vi "Top_Level.vi"() -> ()   [LabVIEW 2013]
uses:
  Classes/OSSP_Problem.lvclass
  Classes/GA.lvclass
  Classes/GA_Class/Controls/Strategy.ctl
  Classes/GA_Class/Controls/Plot Type.ctl
  Classes/GA_Class/Controls/Crossover Type.ctl
  Classes/GA_Class/Controls/Mutation Type.ctl
  Controls/Local Search Type.ctl
  Controls/Problem Instance Type.ctl
  Controls/Scheduler Type.ctl
  Controls/Objective.ctl
  Classes/SA_Class/Controls/Perturbation Method.ctl
  Controls/States.ctl
  Classes/OSSP_Problem.lvclass/OSSP_Problem.ctl
  Classes/GA_Class/Controls/Front Panle Menu.ctl
  Classes/GA.lvclass/GA.ctl
  Controls/SA Solution Selection Method.ctl
  Classes/SA.lvclass/SA.ctl
  Classes/GA_Class/Select Random Solutions.vi
  Classes/GanntChart_Class/Non Delay Scheduler For Tardiness.vi
  Classes/SA_Class/Setters/Write Alpha Value.vi
  Classes/SA_Class/Setters/Write Current Temperature.vi
  Classes/SA_Class/Setters/Write Cooling Strategy.vi
  Classes/SA_Class/Setters/Write Initial Temperature.vi
  Classes/SA_Class/Setters/Write Stop Temperature.vi
  Classes/SA_Class/Setters/Write Cooling Rate.vi
  Classes/SA_Class/Setters/Write Epoch Length.vi
  Classes/SA_Class/Setters/Write Current Solution.vi
  Classes/SA_Class/Setters/Write Best Solution.vi
  Classes/GanntChart_Class/Giffler Thompson Active Schedule Engine.vi
  Classes/GanntChart_Class/Schedule and Create Gannt Chart.vi
  Classes/GanntChart_Class/Calculate Makespan.vi
  Classes/GanntChart_Class/Job Completion Times.vi
  Classes/GanntChart_Class/Reorder Chromosome  After Makespan Calculation.vi
  Classes/SA_Class/Getters/Read Current Solution.vi
  Classes/SA_Class/Setters/Write New Solution.vi
  Classes/SA_Class/Getters/Read New Solution.vi
  Classes/SA_Class/Calculate Acceptance Probability.vi
  Classes/SA_Class/Getters/Read Best Solution.vi
  Classes/SA_Class/Getters/Read Epoch Length.vi
  Classes/SA_Class/Getters/Read Current Temperature.vi
  Classes/SA_Class/Getters/Read Cooling Strategy.vi
  Classes/SA_Class/Getters/Read Cooling Rate.vi
  Classes/SA_Class/Getters/Read Alpha Value.vi
  Classes/SA_Class/Getters/Read Stop Temperature.vi
  Classes/GA_Class/Getters/Read Scheduler.vi
  Classes/GA_Class/Getters/Read Objective .vi
  Classes/GA_Class/Getters/Read Reorder.vi
  Classes/GA_Class/Find Best Solution In Population.vi
  Classes/GanntChart_Class/Operation to Machine Job Tuple.vi
  Classes/GanntChart_Class/Check Other Machines for Schedule Time.vi
  Classes/GanntChart_Class/Schedule Job.vi
  Classes/GanntChart_Class/Find Gaps on Particular Machine.vi
  Classes/GanntChart_Class/Increment Number of Jobs on Machine.vi
  Classes/GanntChart_Class/Find Job On Other Machines.vi
  <vilib>/Analysis/baseanly.llb/Mean (DBL).vi
  Classes/SA_Class/Perturb Current Solution.vi
  Classes/SA.lvclass
  <vilib>/Analysis/NI_AALBase.lvlib
panel:
  out "Makespan":dbl format="%#_13g"
  out "Total Tardiness":i32
  in  "Local Search Per Generation":i32=25
  in  "Perturbation Method":T1
  in  "Local Search":T2
  out "Final Solution":string
  out "Generations":i32(slide) scale=0.0..1001.0
  out "Picture":picture
  in  "Objective":T3=enum."Total Tardiness"
  in  "Reorder":bool=TRUE
  in  "Scheduler":T4=enum."FIFO Scheduler"
  in  "Instance Type":T5=enum."Brucker"
  in  "Mutation Type":T6
  in  "Crossover Type":T7=enum."Linear Order Cx (LOX)"
  in  "Plot Type":T8=enum."Gannt Chart"
  in  "Strategy":T9=enum."Incremental Replacement"
  in  "Number of Generations":i32=1000
  in  "Population Size":u8=30
  in  "Mutation Probability":dbl=0.2
  in  "Crossover Probability":dbl=1.0
  out "Mo4J":u16[][](array[numeric])
  out "JO4M":u16[][](array[numeric])
  out "Due Dates":u16[](array[numeric])
  out "Job Completion Times":u16[](array[numeric])
  out "Job Schedule on Machine":i32[][](array[numeric])
  out "GA.lvclass":refnum<class "GA.lvclass">
  out "OSSP_Problem.lvclass":refnum<class "OSSP_Problem.lvclass">
  out "error out":errorcluster
  in  "error in":errorcluster
  # "Processing tImes =   J1       J2    J3       J4   \n                         M1    X        X      X        X\n                         M2    X        X      X        X\n                         M3    X        X      X        X\n                         M4    X        X      X        X"
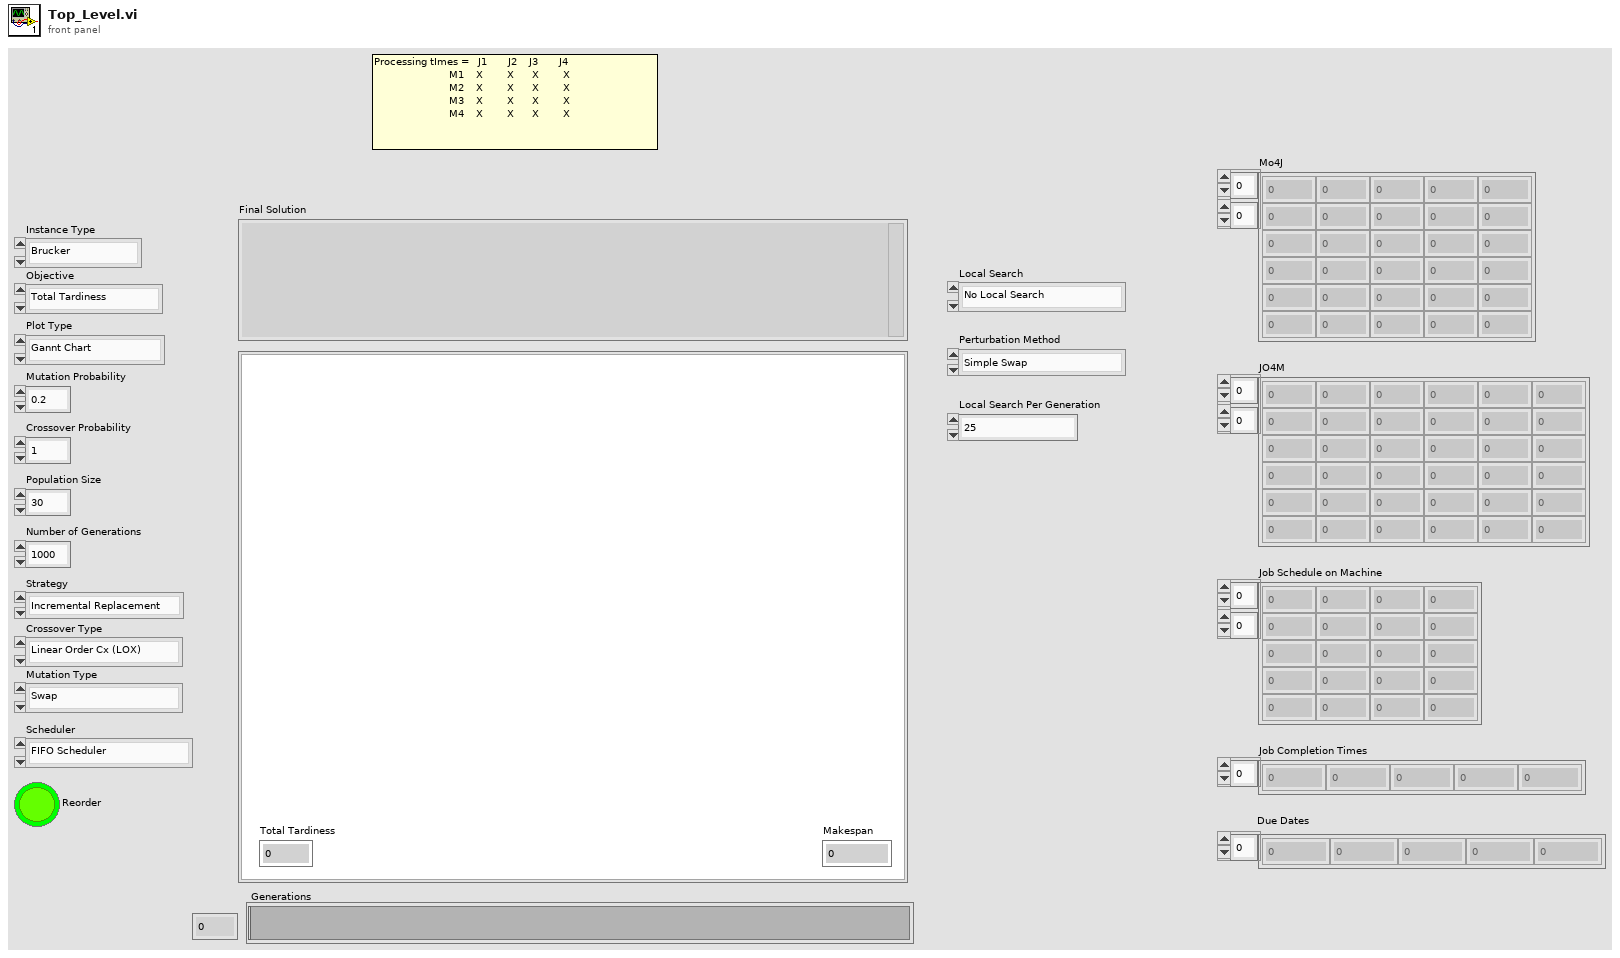
[diagram p1: front panel]
types:
  T1 = typedef "SA.lvclass/Perturbation Method.ctl" = enum16{"Simple Swap", "Insert", "NonRedundantSwap", "Job Order Swap", "Machine Order Swap", "Machine&Job Order Swap", "Critical Path Swap"}
  T2 = typedef "Local Search Type.ctl" = enum16{"No Local Search", "SA Population", "IRH3T(Pop)", "IRH3T(Best Solution)", "SA Best Solution", "SA Random Solution", "SA Random 3 Solutions", "SA Hybrid"}
  T3 = typedef "Objective.ctl" = enum16{"Makespan", "Total Tardiness"}
  T4 = typedef "Scheduler Type.ctl" = enum16{"Non Delay Scheduler", "GT Active Scheduler", "FIFO Scheduler"}
  T5 = typedef "Problem Instance Type.ctl" = enum16{"Taillard", "Gueret-Prins", "Brucker"}
  T6 = typedef "GA.lvclass/Mutation Type.ctl" = enum16{"Swap", "Non-Redundant Swap", "Insert", "Shift", "Shuflle", "Inversion", "SA", "IRH3T", "JO4M Swap", "MO4J Swap", "SPT JO4M", "LCTJ Swap", "ND Mutation"}
  T7 = typedef "GA.lvclass/Crossover Type.ctl" = enum16{"One Point Cx", "Two Point Cx", "Ordered Cx (OX)", "Linear Order Cx (LOX)", "Cycle Cx", "Specialized Cx", "Machine Ass.Uniform Cx", "MPOX1", "MPOX1 Random", "MPOX2", "MPOX2 Random"}
  T8 = typedef "Plot Type.ctl" = enum16{"No Plot", "Min Max Mean Plot", "Gannt Chart"}
  T9 = typedef "Strategy.ctl" = enum16{"Total Replacement", "Incremental Replacement", "Ellitist 1", "Elitist 2", "%10", "%20", "%30", "%40", "%50"}
  T10 = typedef "States.ctl" = enum16{"Read Problem", "Sort Problem", "Calculate Due Dates", "Set Parameters", "Generate Initial Population", "Evaluate Initial Population", "Selection", "Crossover", "Mutation", "Evaluate New Population", "Replace Population with Offspring", "Local Search", "Measure Diversity", "Record Best Solution", "Increment Population Counter", "Show Best Solution", "Plot", "Stop"}
  T11 = typedef "SA Solution Selection Method.ctl" = enum16{"Random Selection", "Tournament Selection"}
  T12 = typedef "Front Panle Menu.ctl" = cluster{"Crossover Probability":dbl, "Mutation Probability":dbl, "Population Size":u8, "Strategy":T9, "Plot Type":T8, "Crossover Type":T7, "Mutation Type":T6, "Scheduler":T4, "Reorder":bool, "Objective ":T3, "Local Search ":T2}
  T13 = typedef "Solution_GA.ctl" = cluster{"Schedule":u16[], "Fitness":u16, "Fitness Valid?":bool}
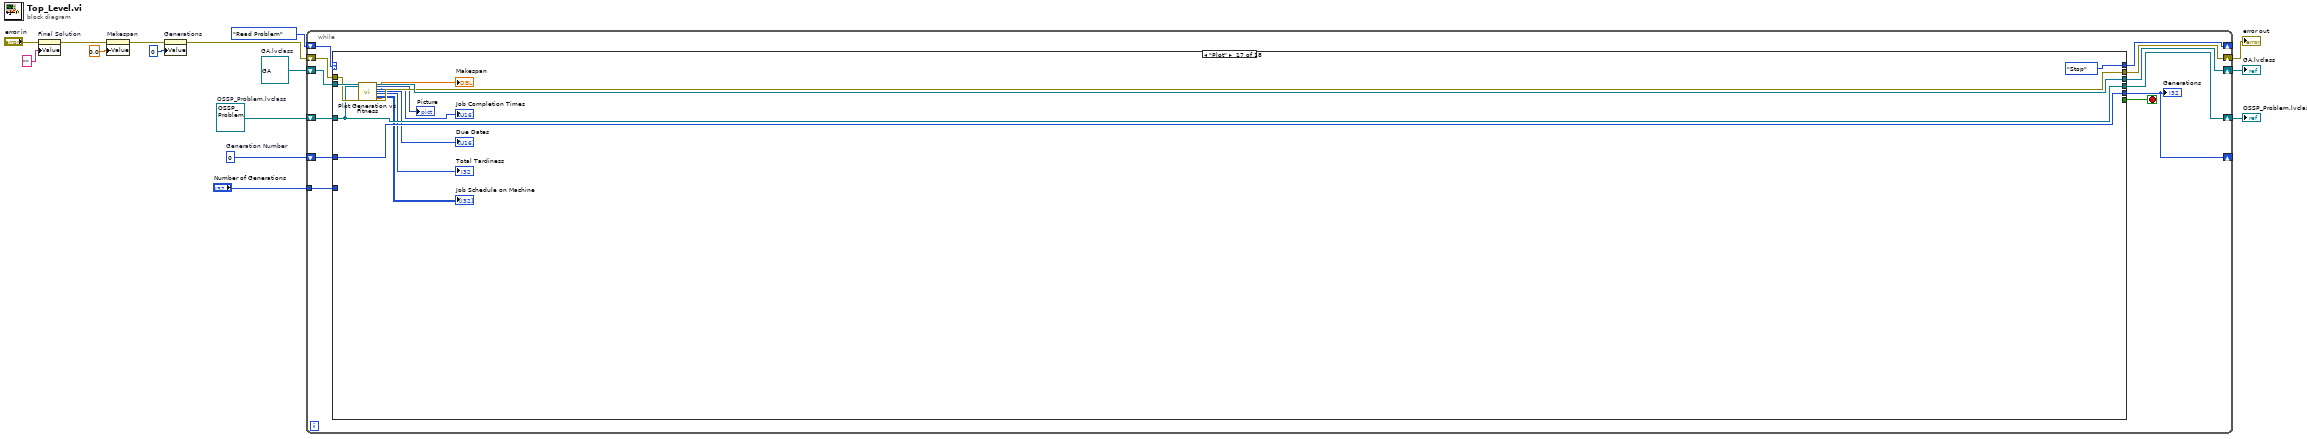
[diagram p0: block diagram]
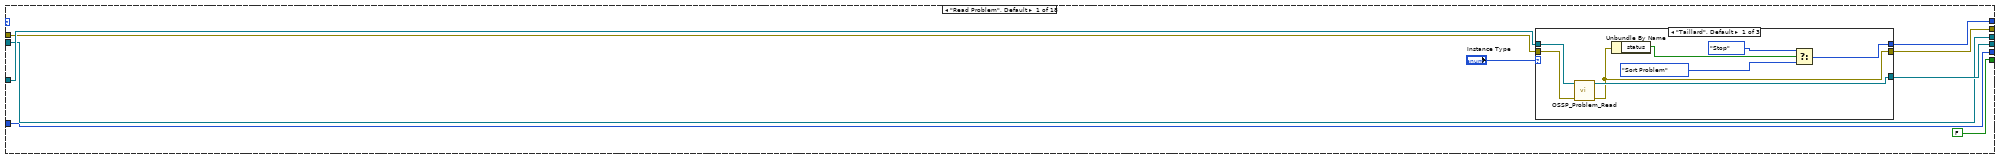
[diagram p2: hidden frame]
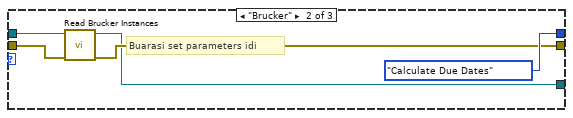
[diagram p3: hidden frame]
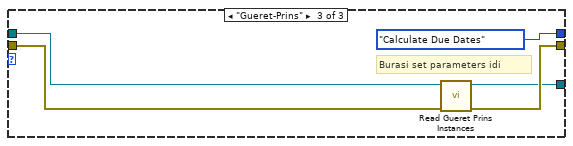
[diagram p4: hidden frame]
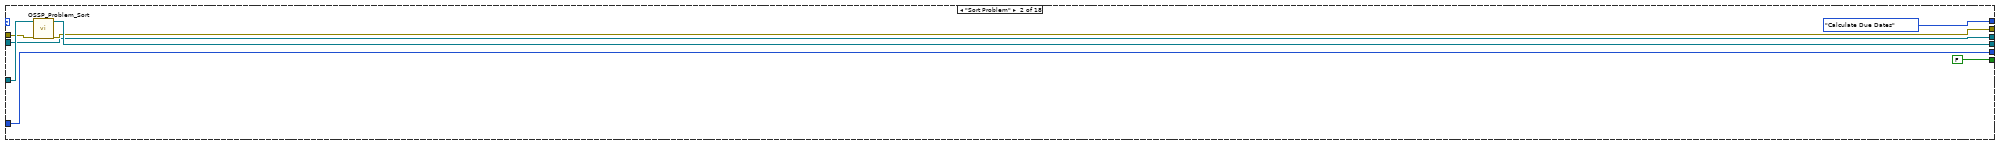
[diagram p5: hidden frame]
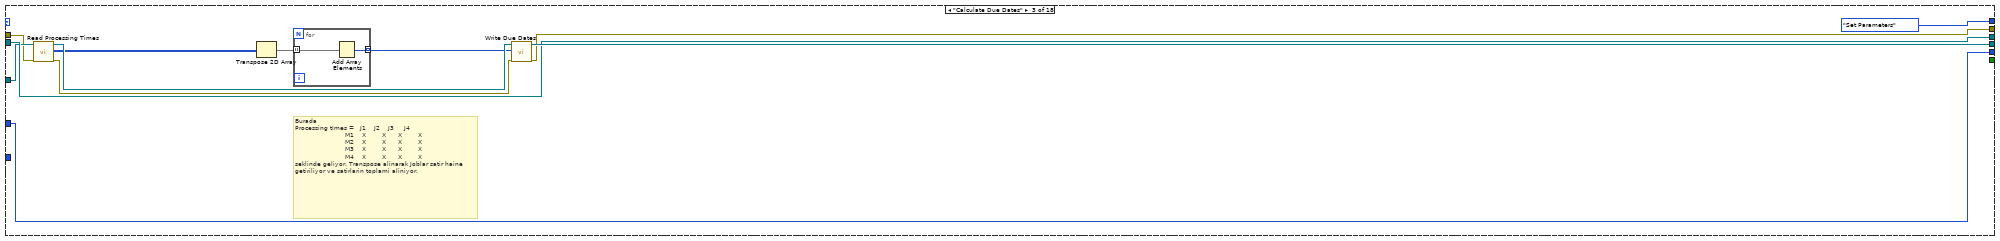
[diagram p6: hidden frame]
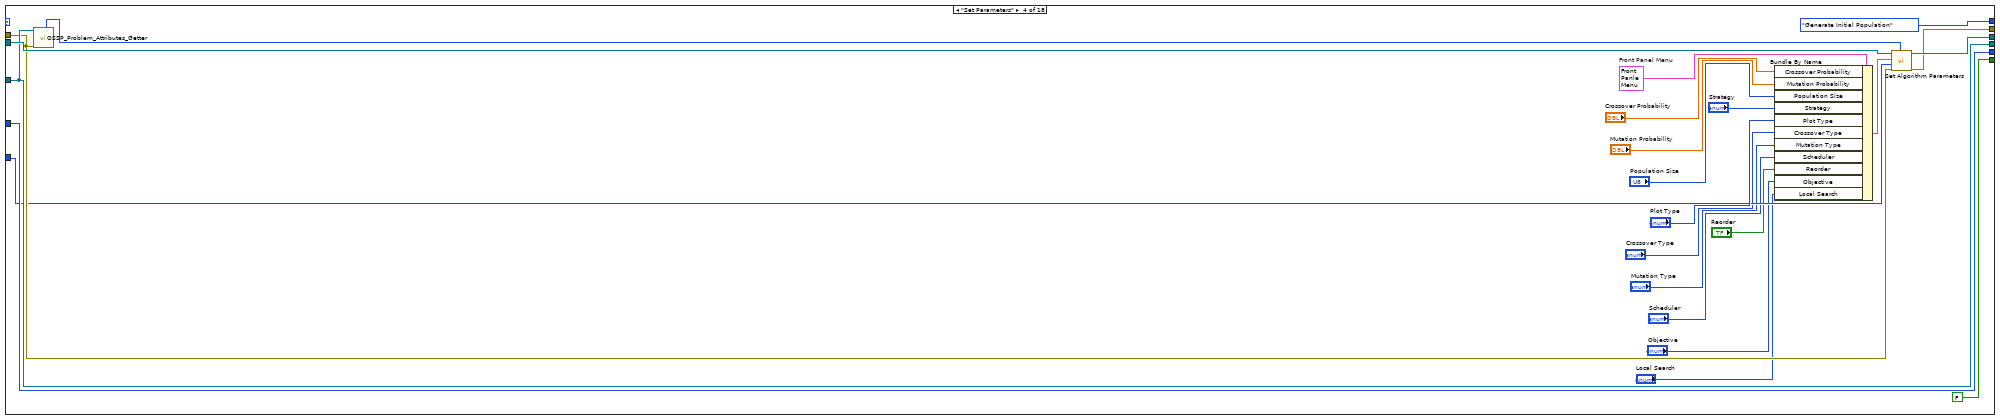
[diagram p7: hidden frame]
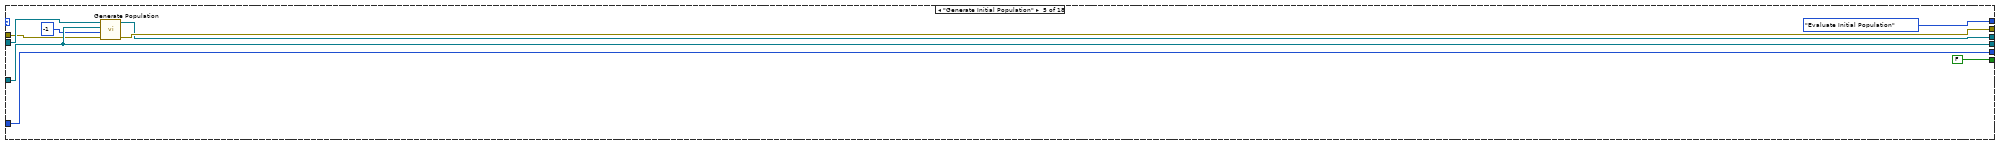
[diagram p8: hidden frame]
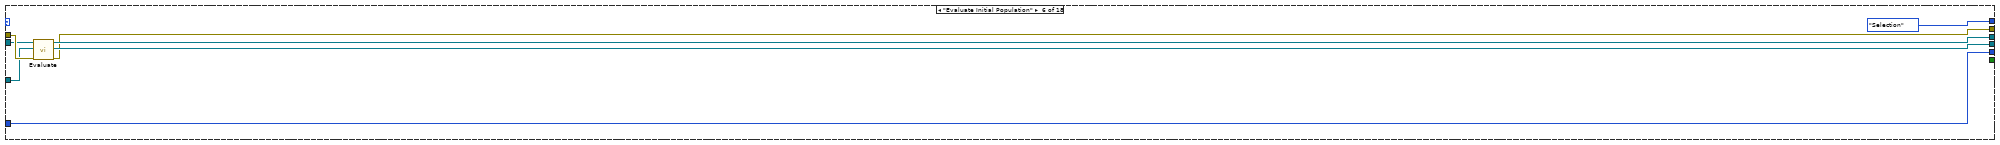
[diagram p9: hidden frame]
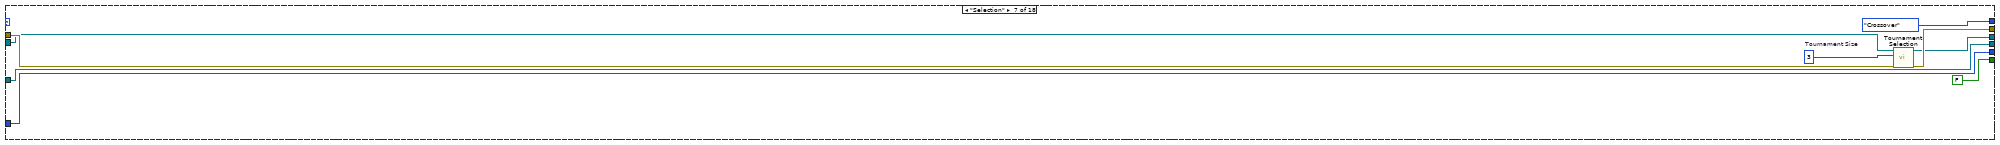
[diagram p10: hidden frame]
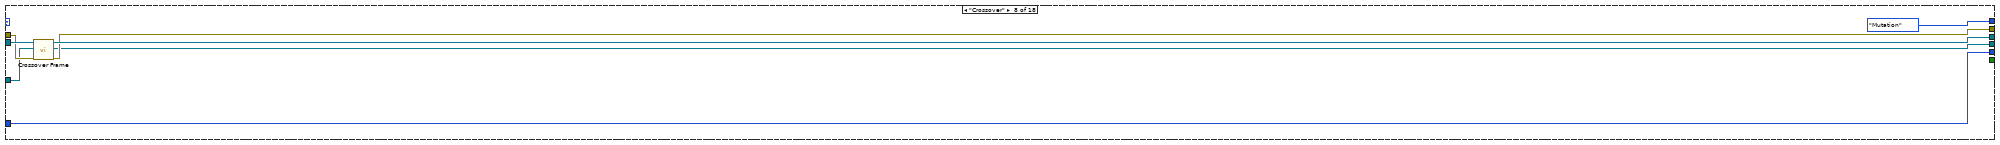
[diagram p11: hidden frame]
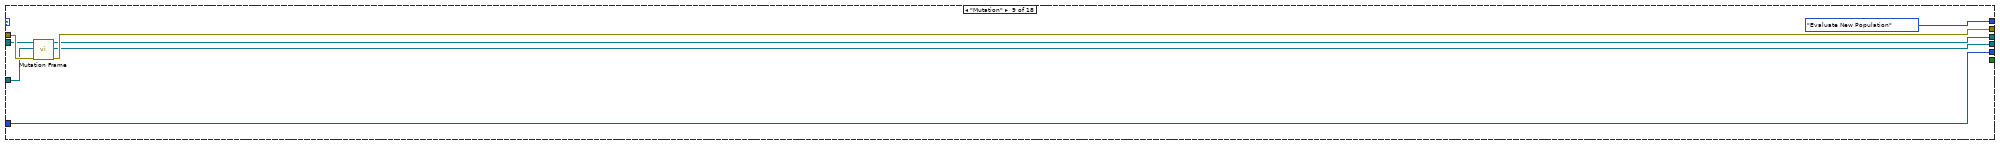
[diagram p12: hidden frame]
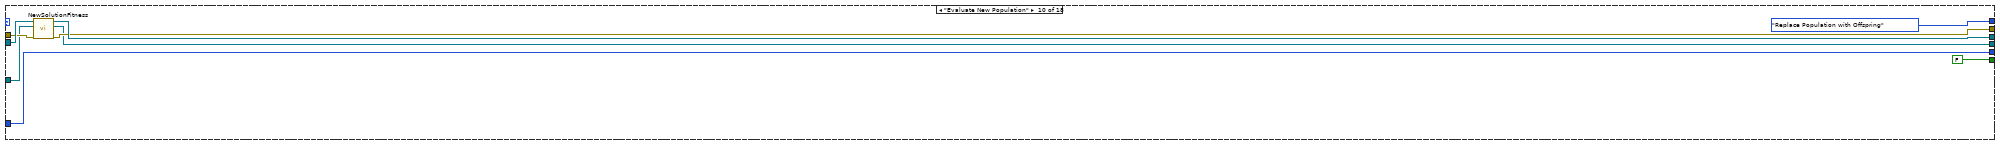
[diagram p13: hidden frame]
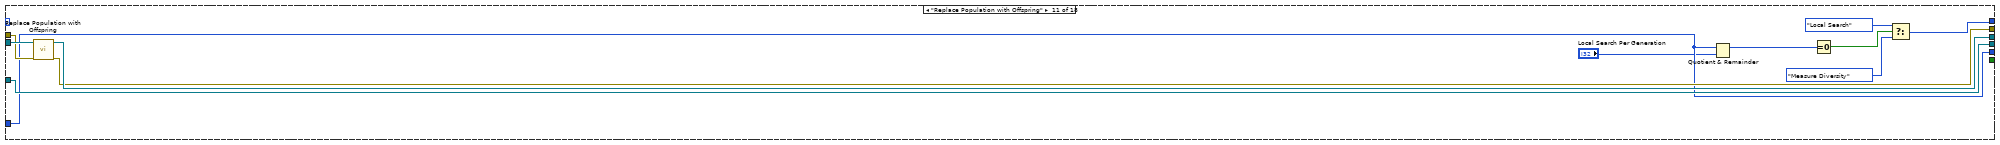
[diagram p14: hidden frame]
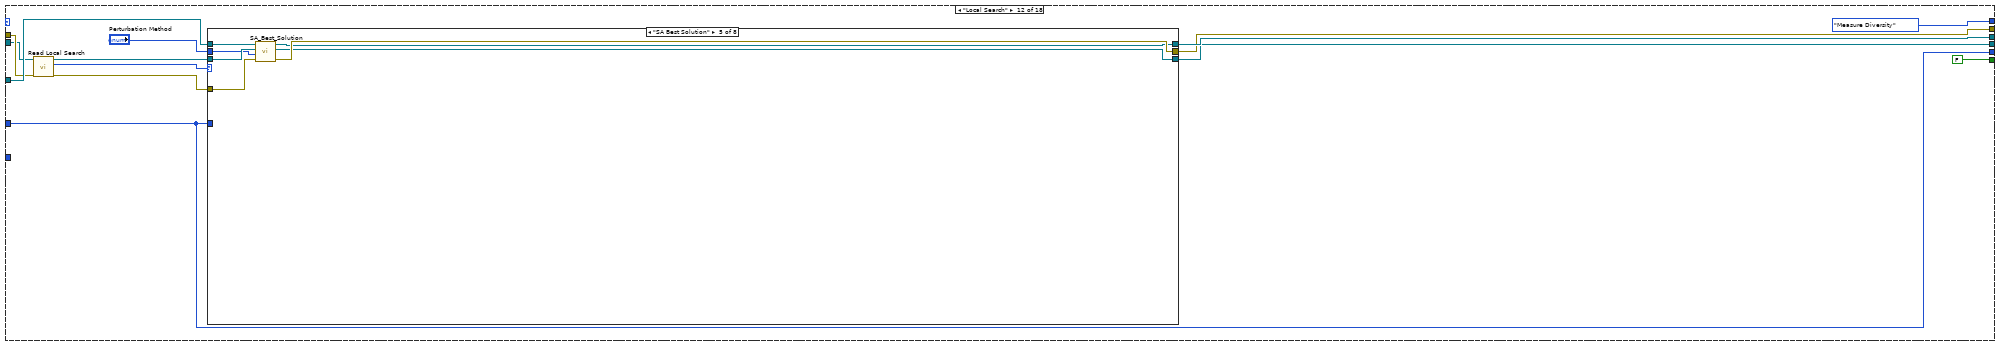
[diagram p15: hidden frame]
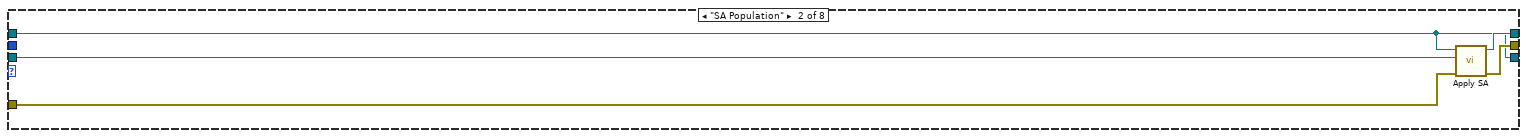
[diagram p17: hidden frame]
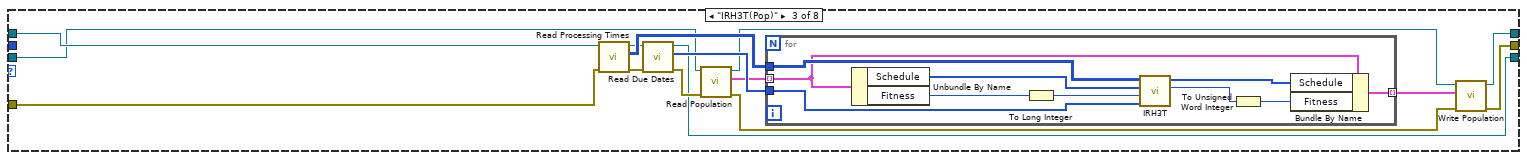
[diagram p18: hidden frame]
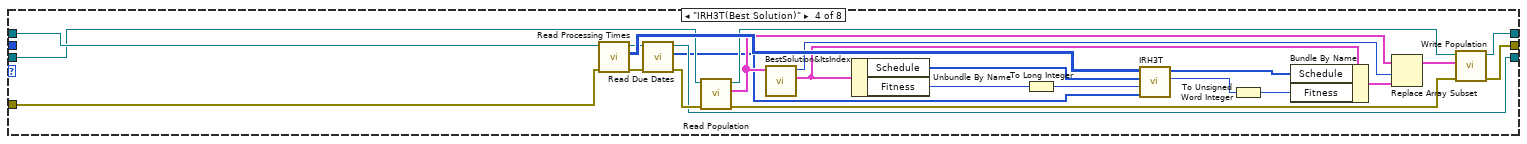
[diagram p19: hidden frame]
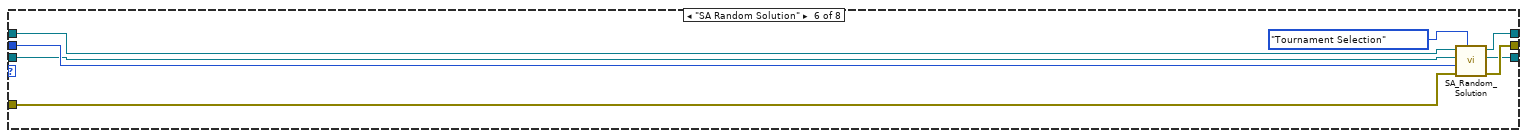
[diagram p20: hidden frame]
diagram:
  w9 = 0  # Generation Number
  w11 = refnum<class "GA.lvclass"> refnum  # GA.lvclass
  w13 = refnum<class "OSSP_Problem.lvclass"> refnum  # OSSP_Problem.lvclass
  n1 = property on="Final Solution" class="Str"(error in="error in", "Value"="" ("Final Solution")) -> (error out=w3:errorcluster)  [unwired: 1 in, 1 out]
  n2 = property on="Makespan" class="DigNum (strict)"(error in=w3, "Value"=0.0 ("Maksepan")) -> (error out=w2:errorcluster)  [unwired: 1 in, 1 out]
  n3 = property on="Generations" class="Slide (strict)"(error in=w2, "Value"=0 ("Generations")) -> (error out=w6:errorcluster)  [unwired: 1 in, 1 out]
  n4 = while {
    shift-right: [w25] -> _
    shift-left: States."Read Problem" -> [w27]
    shift-right: [w23] -> w14
    shift-left: w6 -> [w24]
    shift-right: [w21] -> w12
    shift-left: w13 -> [w22]
    shift-right: [w19] -> w8
    shift-left: w11 -> [w20]
    tunnel: "Number of Generations" -> [w18]
    shift-right: [w16] -> _
    shift-left: w9 -> [w17]
    stop <- w26 stop-if-true
    n5 = case shown="\"Plot\"" w27 {
      tunnel: [FALSE FALSE _ FALSE FALSE _ FALSE _ _ FALSE _ FALSE _ _ _ FALSE _ TRUE] -> w26
      tunnel: [w28 States."Calculate Due Dates" States."Set Parameters" States."Generate Initial Population" States."Evaluate Initial Population" States."Selection" States."Crossover" States."Mutation" States."Evaluate New Population" States."Replace Population with Offspring" w151 States."Measure Diversity" States."Record Best Solution" States."Increment Population Counter" w433 States."Plot" States."Stop" States."Stop"] -> w25
      tunnel: w24 -> [w34 w60 w66 w93 w101 w115 w119 w129 w139 w146 w159 w169 w326 w427 w441 w467 w485 w493]
      tunnel: [w33 w59 w71 w95 w106 w109 w122 w128 w138 w145 w158 w173 w329 w426 w441 w445 w484 w492] -> w23
      tunnel: w22 -> [w35 w62 w68 w94 w102 w113 w125 w127 w135 w144 w162 w175 w330 w431 w440 w457 w483 w495]
      tunnel: [w32 w61 w72 w94 w102 w112 w125 w126 w134 w143 w162 w171 w330 w431 w440 w457 w483 w494] -> w21
      tunnel: w20 -> [w31 w56 w70 w99 w105 w114 w118 w131 w137 w148 w161 w166 w325 w429 w439 w469 w487 w491]
      tunnel: [w31 w56 w70 w98 w104 w110 w117 w130 w136 w147 w160 w174 w328 w428 w439 w468 w486 w491] -> w19
      tunnel: w18 -> [_ _ _ w84 _ _ _ _ _ _ _ _ w322 _ w437 _ _ _]
      tunnel: [w30 w55 w74 w91 w103 w111 w123 w132 w141 w150 w157 w164 w323 w425 w435 w471 w489 w490] -> w16
      tunnel: w17 -> [w30 w55 w74 w91 w103 w111 w123 w132 w141 w150 w157 w164 w324 w425 w438 w471 w489 w490]
      frame "Read Problem", Default {
        n6 = case shown="\"Taillard\", Default" "Instance Type" {
          tunnel: w35 -> [w44 w46 w52]
          tunnel: w34 -> [w43 w48 w54]
          tunnel: [w41 w47 w53] -> w33
          tunnel: [w42 w45 w51] -> w32
          tunnel: [w37 States."Calculate Due Dates" States."Calculate Due Dates"] -> w28
          frame "Taillard", Default {
            n7 = call "OSSP_Problem_Read.vi"("error in (no error)"=w43, "OSSP_Problem.lvclass In"=w44) -> ("error out"=w41:errorcluster, "OSSP_Problem.lvclass Out"=w42:refnum<class "OSSP_Problem.lvclass">)  [unwired: 8 in]
            n8 = Unbundle By Name(w41) -> ("status"=w40:bool)
            n9 = Select(t=States."Stop", s=w40, f=States."Sort Problem") -> (s? t:f=w37:T10)
          }
          frame "Brucker" {
            # "Buarasi set parameters idi"
            n10 = call "Read Brucker Instances.vi"("error in (no error)"=w48, "OSSP_Problem in"=w46) -> ("error out"=w47:errorcluster, "OSSP_Problem out"=w45:refnum<class "OSSP_Problem.lvclass">)  [unwired: 8 in]
          }
          frame "Gueret-Prins" {
            # "Burasi set parameters idi"
            n11 = call "Read Gueret Prins Instances.vi"("error in (no error)"=w54, "OSSP_Problem in"=w52) -> ("error out"=w53:errorcluster, "OSSP_Problem out"=w51:refnum<class "OSSP_Problem.lvclass">)  [unwired: 8 in]
          }
        }
      }
      frame "Sort Problem" {
        n12 = call "OSSP_Problem_Sort.vi"("error in (no error)"=w60, "OSSP_Problem.lvclass In"=w62) -> ("error out"=w59:errorcluster, "OSSP_Problem.lvclass Out"=w61:refnum<class "OSSP_Problem.lvclass">)  [unwired: 8 in]
      }
      frame "Calculate Due Dates" {
        # "Burada \nProcessing tImes =   J1    J2    J3     J4   \n                         M1    X        X      X        X\n                         M2    X        X      X        X\n                         M3    X        X      X        X\n                         M4    X        X      X        X\nseklinde geliyor. Transpose alinarak Joblar satir haine getiriliyor ve satirlarin toplami aliniyor."
        n13 = call-dynamic "Read Processing Times.vi"("error in (no error)"=w66, "OSSP_Problem in"=w68) -> ("error out"=w69:errorcluster, "Processing Times"=w64:u16[][], "OSSP_Problem out"=w67:refnum<class "OSSP_Problem.lvclass">)  [unwired: 7 in]
        n14 = Transpose 2D Array(2D array=w64) -> (transposed array=w65:u16[][])
        n15 = for {
          tunnel: w65 -> [w76] mode=indexing
          tunnel: [w75] -> w63 mode=indexing
          n16 = Add Array Elements(numeric array=w76) -> (sum=w75:u16)
        }
        n17 = call "Write Due Dates.vi"("error in (no error)"=w69, "Due Dates"=w63, "OSSP_Problem in"=w67) -> ("error out"=w71:errorcluster, "OSSP_Problem out"=w72:refnum<class "OSSP_Problem.lvclass">)  [unwired: 7 in]
      }
      frame "Set Parameters" {
        w90 = T12 {"Crossover Probability"=0.75, "Mutation Probability"=0.2, "Population Size"=80, "Strategy"=enum."Total Replacement", "Plot Type"=enum."No Plot", "Crossover Type"=enum."One Point Cx", "Mutation Type"=enum."Swap", "Scheduler"=enum."Non Delay Scheduler", "Reorder"=FALSE, "Objective "=enum."Makespan", "Local Search "=enum."No Local Search"}  # Front Panel Menu
        n18 = call "OSSP_Problem_Attributes_Getter.vi"("error in (no error)"=w93, "OSSP_Problem in"=w94) -> ("Dimension"=w92:i32)  [unwired: 3 in, 6 out]
        n19 = Bundle By Name(cluster=w90, "Crossover Probability"="Crossover Probability", "Mutation Probability"="Mutation Probability", "Population Size"="Population Size", "Strategy"="Strategy", "Plot Type"="Plot Type", "Crossover Type"="Crossover Type", "Mutation Type"="Mutation Type", "Scheduler"="Scheduler", "Reorder"="Reorder", "Objective"="Objective", "Local Search"="Local Search") -> (w83:T12)
        n20 = call "Set Algorithm Parameters.vi"("Dimension"=w92, "error in (no error)"=w93, "Number of Generations"=w84, "Front Panel Menu"=w83, "GA in"=w99) -> ("error out"=w95:errorcluster, "GA out"=w98:refnum<class "GA.lvclass">)  [unwired: 5 in]
      }
      frame "Generate Initial Population" {
        n21 = call "Generate Population.vi"("error in (no error)"=w101, "seed"=-1, "OSSP_Problem.lvclass"=w102, "GA in"=w105) -> ("error out"=w106:errorcluster, "GA out"=w104:refnum<class "GA.lvclass">)  [unwired: 6 in]
      }
      frame "Evaluate Initial Population" {
        n22 = call "Evaluate.vi"("error in (no error)"=w115, "OSSP_Problem.lvclass"=w113, "GA in"=w114) -> ("error out"=w109:errorcluster, "OSSP_Problem out"=w112:refnum<class "OSSP_Problem.lvclass">, "GA out"=w110:refnum<class "GA.lvclass">)  [unwired: 6 in]
      }
      frame "Selection" {
        w121 = 3  # Tournament Size
        n23 = call "Tournament Selection.vi"("error in (no error)"=w119, "Tournament Size"=w121, "GA.lvclass In"=w118) -> ("error out"=w122:errorcluster, "GA.lvclass Out"=w117:refnum<class "GA.lvclass">)  [unwired: 7 in]
      }
      frame "Crossover" {
        n24 = call "Crossover Frame.vi"("error in (no error)"=w129, "OSSP_Problem In"=w127, "GA in"=w131) -> ("error out"=w128:errorcluster, "OSSP_Problem Out"=w126:refnum<class "OSSP_Problem.lvclass">, "GA out"=w130:refnum<class "GA.lvclass">)  [unwired: 6 in]
      }
      frame "Mutation" {
        n25 = call "Mutation Frame.vi"("error in (no error)"=w139, "OSSP_Problem"=w135, "GA in"=w137) -> ("error out"=w138:errorcluster, "OSSP_Problem Out"=w134:refnum<class "OSSP_Problem.lvclass">, "GA out"=w136:refnum<class "GA.lvclass">)  [unwired: 6 in]
      }
      frame "Evaluate New Population" {
        n26 = call "NewSolutionFitness.vi"("error in (no error)"=w146, "OSSP_Problem.lvclass"=w144, "GA in"=w148) -> ("error out"=w145:errorcluster, "OSSP_Problem out"=w143:refnum<class "OSSP_Problem.lvclass">, "GA out"=w147:refnum<class "GA.lvclass">)  [unwired: 6 in]
      }
      frame "Replace Population with Offspring" {
        n27 = call "Replace Population with Offspring.vi"("error in (no error)"=w159, "GA in"=w161) -> ("error out"=w158:errorcluster, "GA out"=w160:refnum<class "GA.lvclass">)  [unwired: 8 in]
        n28 = Quotient & Remainder(x=w157, y="Local Search Per Generation") -> (x-y*floor(x/y)=w155:i32)  [unwired: 1 out]
        n29 = Equal To 0?(x=w155) -> (x = 0?=w154:bool)
        n30 = Select(t=States."Local Search", s=w154, f=States."Measure Diversity") -> (s? t:f=w151:T10)
      }
      frame "Local Search" {
        n31 = call "Read Local Search .vi"("error in (no error)"=w169, "GA in"=w166) -> ("error out"=w168:errorcluster, "Local Search"=w167:T2, "GA out"=w165:refnum<class "GA.lvclass">)  [unwired: 7 in]
        n32 = case shown="\"SA Best Solution\"" w167 {
          tunnel: w165 -> [w177 w183 w192 w221 w239 w241 w288 w306]
          tunnel: w168 -> [w178 w182 w197 w224 w238 w242 w289 w305]
          tunnel: w175 -> [w176 w179 w196 w226 w235 w245 w277 w302]
          tunnel: [w177 w181 w187 w220 w236 w246 w253 w303] -> w174
          tunnel: [w178 w180 w185 w223 w237 w247 w251 w304] -> w173
          tunnel: [w176 w179 w190 w225 w234 w244 w277 w301] -> w171
          tunnel: w164 -> [_ _ _ _ _ _ _ w300]
          tunnel: "Perturbation Method" -> [_ _ _ _ w233 w243 w250 w296]
          frame "No Local Search", Default {
          }
          frame "SA Population" {
            n33 = call "Apply SA.vi"("error in (no error)"=w182, "GA.lvclass"=w183, "OSSP_Problem in"=w179) -> ("error out"=w180:errorcluster, "GA out"=w181:refnum<class "GA.lvclass">)  [unwired: 7 in]
          }
          frame "IRH3T(Pop)" {
            n34 = call-dynamic "Read Processing Times.vi"("error in (no error)"=w197, "OSSP_Problem in"=w196) -> ("error out"=w194:errorcluster, "Processing Times"=w198:u16[][], "OSSP_Problem out"=w195:refnum<class "OSSP_Problem.lvclass">)  [unwired: 7 in]
            n35 = call "Read Due Dates.vi"("error in (no error)"=w194, "OSSP_Problem in"=w195) -> ("error out"=w191:errorcluster, "Due Dates"=w193:u16[], "OSSP_Problem out"=w190:refnum<class "OSSP_Problem.lvclass">)  [unwired: 7 in]
            n36 = call-dynamic "Read Population.vi"("error in (no error)"=w191, "GA in"=w192) -> ("error out"=w186:errorcluster, "Population"=w189:T13[], "GA out"=w188:refnum<class "GA.lvclass">)  [unwired: 7 in]
            n37 = for {
              tunnel: w198 -> [w208]
              tunnel: w193 -> [w199]
              tunnel: w189 -> [w207] mode=indexing
              tunnel: [w206] -> w184 mode=indexing
              n38 = Unbundle By Name(w207) -> ("Schedule"=w204:u16[], "Fitness"=w203:u16)
              n39 = To Long Integer(number=w203) -> (32bit integer=w202:i32)
              n40 = call "IRH3T.vi"("Due Dates"=w199, "Initial Tardiness"=w202, "Schedule 2B Improved"=w204, "Proocessing Times  (Machines x Jobs)"=w208) -> ("Total Tardiness"=w201:i32, "IRH3T (Reordered) Schedule Out"=w205:u16[])  [unwired: 6 in]
              n41 = To Unsigned Word Integer(number=w201) -> (unsigned 16bit integer=w200:u16)
              n42 = Bundle By Name(cluster=w207, "Schedule"=w205, "Fitness"=w200) -> (w206:T13)
            }
            n43 = call "Write Population.vi"("error in (no error)"=w186, "Population"=w184, "GA in"=w188) -> ("error out"=w185:errorcluster, "GA out"=w187:refnum<class "GA.lvclass">)  [unwired: 7 in]
          }
          frame "IRH3T(Best Solution)" {
            n44 = call-dynamic "Read Processing Times.vi"("error in (no error)"=w224, "OSSP_Problem in"=w226) -> ("error out"=w230:errorcluster, "Processing Times"=w232:u16[][], "OSSP_Problem out"=w231:refnum<class "OSSP_Problem.lvclass">)  [unwired: 7 in]
            n45 = call "Read Due Dates.vi"("error in (no error)"=w230, "OSSP_Problem in"=w231) -> ("error out"=w229:errorcluster, "Due Dates"=w211:u16[], "OSSP_Problem out"=w225:refnum<class "OSSP_Problem.lvclass">)  [unwired: 7 in]
            n46 = call-dynamic "Read Population.vi"("error in (no error)"=w229, "GA in"=w221) -> ("error out"=w227:errorcluster, "Population"=w218:T13[], "GA out"=w228:refnum<class "GA.lvclass">)  [unwired: 7 in]
            n47 = call "BestSolution&ItsIndex.vi"("Population"=w218) -> ("Best Solution In the Population"=w219:T13, "Best Solution Index for Replace"=w217:i32)  [unwired: 9 in]
            n48 = Unbundle By Name(w219) -> ("Schedule"=w214:u16[], "Fitness"=w213:u16)
            n49 = To Long Integer(number=w213) -> (32bit integer=w212:i32)
            n50 = call "IRH3T.vi"("Due Dates"=w211, "Initial Tardiness"=w212, "Schedule 2B Improved"=w214, "Proocessing Times  (Machines x Jobs)"=w232) -> ("Total Tardiness"=w210:i32, "IRH3T (Reordered) Schedule Out"=w222:u16[])  [unwired: 6 in]
            n51 = To Unsigned Word Integer(number=w210) -> (unsigned 16bit integer=w209:u16)
            n52 = Bundle By Name(cluster=w219, "Schedule"=w222, "Fitness"=w209) -> (w216:T13)
            n53 = Replace Array Subset(array=w218, new element=w216, index=w217) -> (w215:T13[])
            n54 = call "Write Population.vi"("error in (no error)"=w227, "Population"=w215, "GA in"=w228) -> ("error out"=w223:errorcluster, "GA out"=w220:refnum<class "GA.lvclass">)  [unwired: 7 in]
          }
          frame "SA Best Solution" {
            n55 = call "SA_Best_Solution.vi"("error in (no error)"=w238, "Perturbation Method"=w233, "GA.lvclass"=w239, "OSSP_Problem in"=w235) -> ("error out"=w237:errorcluster, "OSSP_Problem out"=w234:refnum<class "OSSP_Problem.lvclass">, "GA out"=w236:refnum<class "GA.lvclass">)  [unwired: 5 in]
          }
          frame "SA Random Solution" {
            n56 = call "SA_Random_Solution.vi"("Selection Method"=SA_Solution_Selection_Method."Tournament Selection", "error in (no error)"=w242, "Perturbation Method"=w243, "GA.lvclass"=w241, "OSSP_Problem in"=w245) -> ("error out"=w247:errorcluster, "OSSP_Problem out"=w244:refnum<class "OSSP_Problem.lvclass">, "GA out"=w246:refnum<class "GA.lvclass">)  [unwired: 4 in]
          }
          frame "SA Random 3 Solutions" {
            # "Machine"
            n57 = call-dynamic "Read Population.vi"("error in (no error)"=w289, "GA in"=w288) -> ("error out"=w290:errorcluster, "Population"=w273:T13[], "GA out"=w254:refnum<class "GA.lvclass">)  [unwired: 7 in]
            n58 = Array Size(array=w273) -> (size(s)=w285:i32)
            n59 = for {
              N: 3 -> [_]
              tunnel: w285 -> [w292]
              tunnel: [w291] -> w286 mode=indexing
              n60 = Random Number (0-1)() -> (number: 0 to 1=w295:dbl)
              n61 = Multiply(x=w295, y=w292) -> (x*y=w294:dbl)
              n62 = Round Toward -Infinity(1:w294) -> (0:w293:dbl)
              n63 = To Unsigned Byte Integer(number=w293) -> (unsigned 8bit integer=w291:u8)
            }
            n64 = call "Remove Duplicates In Array.vi"("Max Index Bound"=w285, "Random Numbers Array"=w286) -> ("Random Numbers Array without Duplicates"=w284:i32[])  [unwired: 9 in]
            n65 = Index Array(array=w284, index #1=0 ("index"), index #2=1 ("index"), index #3=2 ("index")) -> (element #1=w262:i32, element #2=w261:i32, element #3=w260:i32)
            n66 = Index Array(array=w273, index #1=w262, index #2=w261, index #3=w260) -> (element #1=w272:T13, element #2=w268:T13, element #3=w259:T13)
            n67 = Unbundle By Name(w272) -> ("Schedule"=w280:u16[])
            n68 = Unbundle By Name(w268) -> ("Schedule"=w279:u16[])
            n69 = Unbundle By Name(w259) -> ("Schedule"=w278:u16[])
            n70 = call "SA_Selected_Solution.vi"("Perturbation Method"=w250, "error in (no error)"=w290, "Schedule In"=w280, "GA.lvclass"=w254, "OSSP_Problem in"=w277) -> ("error out"=w276:errorcluster, "Schedule Out"=w271:u16[], "Fitness"=w270:i16)  [unwired: 2 in, 2 out]
            n71 = call "SA_Selected_Solution.vi"("Perturbation Method"=w250, "error in (no error)"=w290, "Schedule In"=w279, "GA.lvclass"=w254, "OSSP_Problem in"=w277) -> ("error out"=w275:errorcluster, "Schedule Out"=w267:u16[], "Fitness"=w266:i16)  [unwired: 2 in, 2 out]
            n72 = call "SA_Selected_Solution.vi"("Perturbation Method"=w250, "error in (no error)"=w290, "Schedule In"=w278, "GA.lvclass"=w254, "OSSP_Problem in"=w277) -> ("error out"=w274:errorcluster, "Schedule Out"=w257:u16[], "Fitness"=w256:i16)  [unwired: 2 in, 2 out]
            n73 = Merge Errors(w276, w275, w274) -> (w252:errorcluster)
            n74 = Bundle By Name(cluster=w272, "Schedule"=w271, "Fitness"=w270, "Fitness Valid?"=TRUE) -> (w269:T13)
            n75 = Bundle By Name(cluster=w268, "Schedule"=w267, "Fitness"=w266, "Fitness Valid?"=TRUE) -> (w263:T13)
            n76 = Bundle By Name(cluster=w259, "Schedule"=w257, "Fitness"=w256, "Fitness Valid?"=TRUE) -> (w258:T13)
            n77 = Replace Array Subset(array=w273, new element #1=w269, index #1=w262, new element #2=w263, index #2=w261, new element #3=w258, index #3=w260) -> (w249:T13[])
            n78 = call "Sort Population In Descending Order.vi"("Population"=w249) -> ("Population In Descending Order"=w248:T13[])  [unwired: 9 in, 1 out]
            n79 = call "Write Population.vi"("error in (no error)"=w252, "Population"=w248, "GA in"=w254) -> ("error out"=w251:errorcluster, "GA out"=w253:refnum<class "GA.lvclass">)  [unwired: 7 in]
          }
          frame "SA Hybrid" {
            n80 = Quotient & Remainder(x=w300, y=2) -> (x-y*floor(x/y)=w298:i32)  [unwired: 1 out]
            n81 = Equal To 0?(x=w298) -> (x = 0?=w297:bool)
            n82 = case shown="False" w297 {
              tunnel: w306 -> [w314 w321]
              tunnel: w305 -> [w310 w320]
              tunnel: [w309 w319] -> w304
              tunnel: [w311 w318] -> w303
              tunnel: w302 -> [w313 w317]
              tunnel: [w312 w316] -> w301
              tunnel: w296 -> [w308 w315]
              frame False {
                n83 = call "SA_Random_Solution.vi"("Selection Method"=SA_Solution_Selection_Method."Tournament Selection", "error in (no error)"=w310, "Perturbation Method"=w308, "GA.lvclass"=w314, "OSSP_Problem in"=w313) -> ("error out"=w309:errorcluster, "OSSP_Problem out"=w312:refnum<class "OSSP_Problem.lvclass">, "GA out"=w311:refnum<class "GA.lvclass">)  [unwired: 4 in]
              }
              frame True {
                n84 = call "SA_Best_Solution.vi"("error in (no error)"=w320, "Perturbation Method"=w315, "GA.lvclass"=w321, "OSSP_Problem in"=w317) -> ("error out"=w319:errorcluster, "OSSP_Problem out"=w316:refnum<class "OSSP_Problem.lvclass">, "GA out"=w318:refnum<class "GA.lvclass">)  [unwired: 5 in]
              }
            }
          }
        }
      }
      frame "Measure Diversity" {
        n85 = disable-structure shown="Enabled" {
          disable-tunnel: [w344 w371 w374] -> w329
          disable-tunnel: [w343 w370 w372] -> w328
          disable-tunnel: w326 -> [w341 w371 w387]
          disable-tunnel: w325 -> [w339 w370 w386]
          disable-tunnel: w324 -> [_ w369 w389]
          disable-tunnel: [_ w369 w389] -> w323
          disable-tunnel: w322 -> [_ _ w388]
          frame Disabled {
            n86 = call "Read Population Size.vi"("error in (no error)"=w341, "GA in"=w339) -> ("error out"=w340:errorcluster, "Population Size"=w334:u8, "GA out"=w338:refnum<class "GA.lvclass">)  [unwired: 7 in]
            n87 = call "Calculate Entropy.vi"("error in (no error)"=w340, "GA in"=w339) -> ("error out"=w342:errorcluster, "Unique Fitness Values"=w332:i32)  [unwired: 7 in, 1 out]
            n88 = To Double Precision Float(number=w334) -> (double precision float=w333:dbl)
            n89 = To Double Precision Float(number=w332) -> (double precision float=w331:dbl)
            n90 = Divide(x=w333, y=2.0) -> (x/y=w336:dbl)
            n91 = Less?(x=w331, y=w336) -> (x < y?=w335:bool)
            n92 = case shown="True" w335 {
              tunnel: w342 -> [w345 w360]
              tunnel: [w345 w347] -> w344
              tunnel: w338 -> [w346 w359]
              tunnel: [w346 w349] -> w343
              frame False {
              }
              frame True {
                n93 = Random Number (0-1)() -> (number: 0 to 1=w368:dbl)
                n94 = Multiply(x=w368, y=100.0) -> (x*y=w366:dbl)
                n95 = Random Number (0-1)() -> (number: 0 to 1=w355:dbl)
                n96 = Multiply(x=w355, y=100.0) -> (x*y=w357:dbl)
                n97 = Greater?(x=w366, y=30.0) -> (0:w364:bool)
                n98 = Select(t=Crossover_Type."One Point Cx" ("Crossover Type"), s=w364, f=Crossover_Type."Ordered Cx (OX)" ("Crossover Type")) -> (s? t:f=w361:T7)
                n99 = Greater?(x=w357, y=40.0) -> (0:w351:bool)
                n100 = Select(t=Mutation_Type."Swap" ("Mutation Type"), s=w351, f=Mutation_Type."Insert") -> (s? t:f=w353:T6)
                n101 = call "Write Crossover Type.vi"("error in (no error)"=w360, "Crossover Type"=w361, "GA in"=w359) -> ("error out"=w348:errorcluster, "GA out"=w350:refnum<class "GA.lvclass">)  [unwired: 7 in]
                n102 = call "Write Mutation Type.vi"("error in (no error)"=w348, "Mutation Type"=w353, "GA in"=w350) -> ("error out"=w347:errorcluster, "GA out"=w349:refnum<class "GA.lvclass">)  [unwired: 7 in]
              }
            }
          }
          frame Enabled {
          }
          frame Disabled {
            n103 = disable-structure shown="Enabled" {
              disable-tunnel: w389 -> [w399 _]
              disable-tunnel: w388 -> [w398 _]
              disable-tunnel: w387 -> [w397 w407]
              disable-tunnel: w386 -> [w396 w408]
              disable-tunnel: [w391 w407] -> w384
              disable-tunnel: [w390 w408] -> w383
              frame Disabled {
                # "Burada Prins uyguladigi gibi mean tardiness/min tardiness 1.02nin altina inince mutasyonu olasligini degistiren bir fonksiyon yaz"
                n104 = Divide(x=w398, y=50) -> (x/y=w394:dbl)
                n105 = To Long Integer(number=w394) -> (32bit integer=w393:i32)
                n106 = Greater?(x=w399, y=w393) -> (0:w392:bool)
                n107 = case shown="True" w392 {
                  tunnel: w396 -> [w400 w406]
                  tunnel: w397 -> [w401 w405]
                  tunnel: [w401 w404] -> w391
                  tunnel: [w400 w403] -> w390
                  frame False {
                  }
                  frame True {
                    n108 = call "Write Scheduler.vi"("error in (no error)"=w405, "Scheduler"=Scheduler_Type."FIFO Scheduler", "GA in"=w406) -> ("error out"=w404:errorcluster, "GA out"=w403:refnum<class "GA.lvclass">)  [unwired: 7 in]
                  }
                }
              }
              frame Enabled {
              }
            }
            n109 = call-dynamic "Read Population.vi"("error in (no error)"=w384, "GA in"=w383) -> ("error out"=w375:errorcluster, "Population"=w385:T13[], "GA out"=w373:refnum<class "GA.lvclass">)  [unwired: 7 in]
            n110 = for {
              tunnel: w385 -> [w424] mode=indexing
              tunnel: [w423] -> w382 mode=indexing
              n111 = Unbundle By Name(w424) -> ("Fitness"=w423:u16)
            }
            n112 = To Double Precision Float(number=w382) -> (double precision float=w381:dbl[])
            n113 = call-poly <vilib>:"Mean.vi"("X"=w381) -> ("mean"=w380:dbl)  [unwired: 1 out]
            n114 = Array Max & Min(array=w381) -> (min value=w379:dbl)  [unwired: 3 out]
            n115 = Divide(x=w380, y=w379) -> (x/y=w378:dbl)
            n116 = Less Or Equal?(x=w378, y=4.0) -> (x <= y?=w376:bool)
            n117 = case shown="False" w376 {
              tunnel: w373 -> [w417 w422]
              tunnel: w375 -> [w414 w421]
              tunnel: [w412 w420] -> w374
              tunnel: [w415 w419] -> w372
              frame False {
                n118 = call "Read Mutation Probability.vi"("error in (no error)"=w414, "GA in"=w417) -> ("error out"=w413:errorcluster, "Mutation Probability"=w411:dbl, "GA out"=w416:refnum<class "GA.lvclass">)  [unwired: 7 in]
                n119 = Multiply(x=w411, y=0.99) -> (x*y=w409:dbl)
                n120 = call "Write Mutation Probability.vi"("error in (no error)"=w413, "Mutation Probability"=w409, "GA in"=w416) -> ("error out"=w412:errorcluster, "GA out"=w415:refnum<class "GA.lvclass">)  [unwired: 7 in]
              }
              frame True {
                n121 = call "Write Mutation Probability.vi"("error in (no error)"=w421, "Mutation Probability"=0.8, "GA in"=w422) -> ("error out"=w420:errorcluster, "GA out"=w419:refnum<class "GA.lvclass">)  [unwired: 7 in]
              }
            }
          }
        }
      }
      frame "Record Best Solution" {
        n122 = call "Best Solution In Population.vi"("error in (no error)"=w427, "Generation Number"=w425, "GA in"=w429) -> ("error out"=w426:errorcluster, "GA out"=w428:refnum<class "GA.lvclass">)  [unwired: 7 in]
      }
      frame "Increment Population Counter" {
        n123 = Increment(x=w438) -> (x+1=w435:i32)
        n124 = Greater?(x=w435, y=w437) -> (0:w436:bool)
        n125 = Select(t=States."Show Best Solution", s=w436, f=States."Selection") -> (s? t:f=w433:T10)
      }
      frame "Show Best Solution" {
        w451 = "\r"
        n126 = call-dynamic "Read Best Solution Array.vi"("error in (no error)"=w467, "GA in"=w469) -> ("error out"=w447:errorcluster, "Best Solution Array"=w466:T13[], "GA out"=w468:refnum<class "GA.lvclass">)  [unwired: 7 in]
        n127 = call "Find Best Solution In Best Solutions Array.vi"("Best Solution Array"=w466) -> ("Best Solution"=w465:T13)  [unwired: 10 in]
        n128 = call "OSSP_Problem_Attributes_Getter.vi"("error in (no error)"=w447, "OSSP_Problem in"=w457) -> ("OSSP_Problem out"=w450:refnum<class "OSSP_Problem.lvclass">, "Instance"=w453:u8, "Filename"=w455:string)  [unwired: 3 in, 4 out]
        n129 = Unbundle By Name(w465) -> ("Schedule"=w449:u16[], "Fitness"=w463:u16)
        n130 = call-dynamic "Read Number of Machines.vi"("error in (no error)"=w447, "OSSP_Problem in"=w450) -> ("error out"=w446:errorcluster, "Number of Machines"=w448:i32, "OSSP_Problem out"=w444:refnum<class "OSSP_Problem.lvclass">)  [unwired: 7 in]
        n131 = for {
          tunnel: w449 -> [w476] mode=indexing
          shift-right: [w472] -> w462
          shift-left: "Best Sequence = " -> [w475]
          n132 = Number To Decimal String(number=w476) -> (decimal integer string=w474:string)  [unwired: 1 in]
          n133 = call <vilib>:"Space Constant.vi"() -> ("String"=w473:string)
          n134 = Concatenate Strings(w475, w474, w473) -> (w472:string)
        }
        n135 = call "RetrieveJobAndMachineOrders.vi"("error in (no error)"=w446, "Number of Machines"=w448, "Schedule"=w449, "OSSP_Problem in"=w444) -> ("error out"=w445:errorcluster, "Mo4J"=→"Mo4J":u16[][], "JO4M"=→"JO4M":u16[][])  [unwired: 5 in]
        n136 = Number To Decimal String(number=w463) -> (decimal integer string=w461:string)  [unwired: 1 in]
        n137 = Number To Decimal String(number=w453) -> (decimal integer string=w452:string)  [unwired: 1 in]
        n138 = Concatenate Strings(w462, w451, w451, "Fitness = " ("string"), w461, w451, w451, "Filename = " ("string"), w455, w451, "Instance = " ("string"), w452) -> (→"Final Solution":string)
      }
      frame "Plot" {
        n139 = call "Plot Generation vs Fitness.vi"("GA in"=w487, "OSSP_Problem.lvclass"=w483, "error in (no error)"=w485) -> ("GA out"=w486:refnum<class "GA.lvclass">, "Picture"=→"Picture":picture, "Job Completion Times"=→"Job Completion Times":u16[], "Due Dates"=→"Due Dates":u16[], "Total Tardiness"=→"Total Tardiness":i32, "Job Schedule on Machine"=→"Job Schedule on Machine":i32[][], "Maksepan"=→"Makespan":dbl, "error out"=w484:errorcluster)  [unwired: 17 in]
      }
      frame "Stop" {
        n140 = disable-structure shown="Enabled" {
          disable-tunnel: w495 -> [w501 w503]
          disable-tunnel: [w500 w503] -> w494
          disable-tunnel: w493 -> [w499 w502]
          disable-tunnel: [w498 w502] -> w492
          frame Disabled {
            n141 = call "OSSP_Problem_Attributes_Getter.vi"("error in (no error)"=w499, "OSSP_Problem in"=w501) -> ("error out"=w498:errorcluster, "OSSP_Problem out"=w500:refnum<class "OSSP_Problem.lvclass">)  [unwired: 3 in, 5 out]
          }
          frame Enabled {
          }
        }
      }
    }
    "Generations" <- w16
  }
  "error out" <- w14
  "OSSP_Problem.lvclass" <- w12
  "GA.lvclass" <- w8
